vi "Copy .LLB to NI VeriStand dir.vi"(5 "Files Generated by Build":path[](array[path]), 6 "Top Level/Always Included VIs":path[](array[path]), 7 "Destination Path":path, 8 "error in (no error)":errorcluster, 9 "Target Name":string, 10 "Build Specification Name":string, 11 "Project Path":path) -> (0 "error out":errorcluster)   [LabVIEW 2017]
doc: "This VI is called after each run of a build specification. The VI will copy the generated LLB (Engine or System Explorer) into the VeriStand Custom Device folder (...\\Documents\\National Instruments\\NI VeriStand 2013...)."
uses:
  <vilib>/Utility/sysdir.llb/System Directory Type.ctl
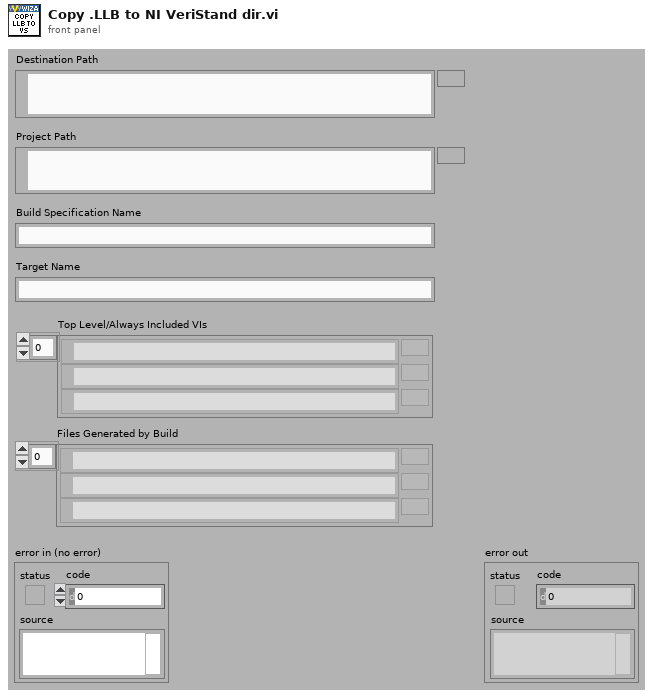
[diagram p1: front panel]
types:
  T1 = typedef "System Directory Type.ctl" = i32
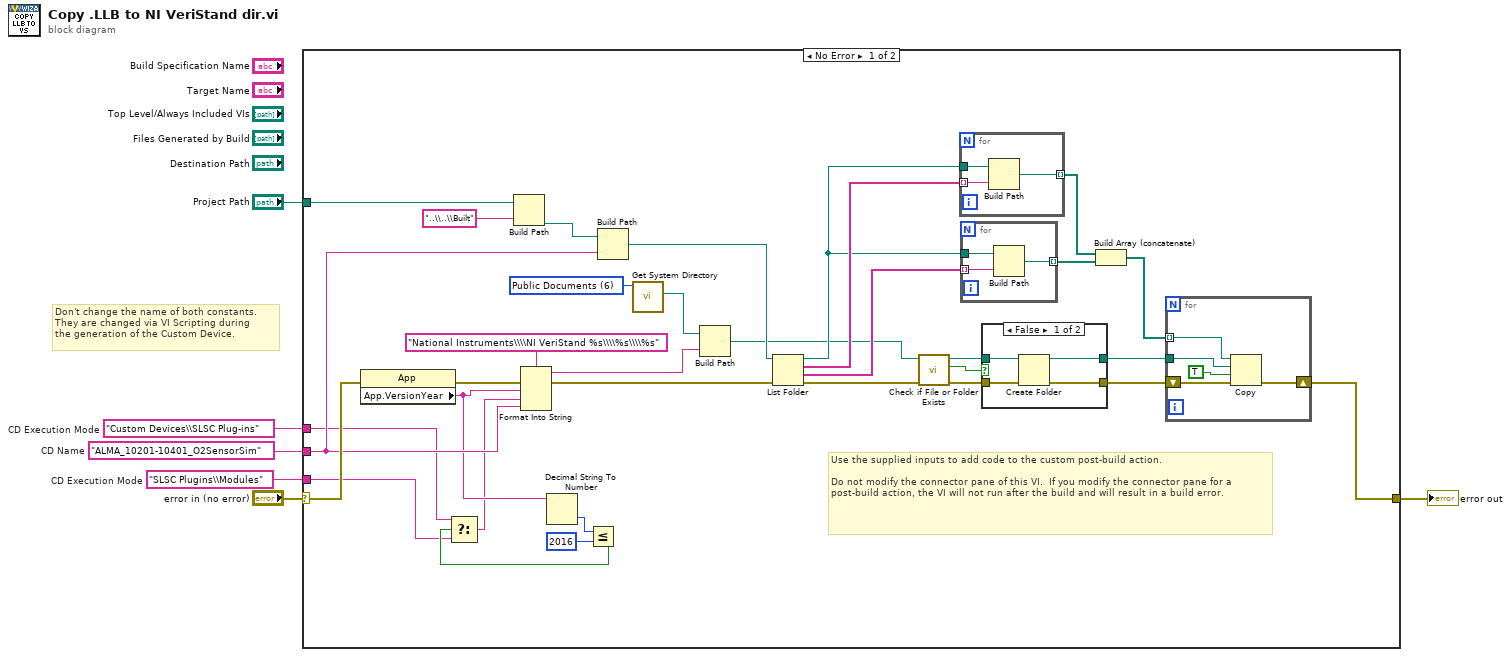
[diagram p0: block diagram]
diagram:
  w1 = "SLSC Plugins\\Modules"  # CD Execution Mode
  w3 = "ALMA_10201-10401_O2SensorSim"  # CD Name
  w4 = "Custom Devices\\SLSC Plug-ins"  # CD Execution Mode
  # "Don't change the name of both constants.\nThey are changed via VI Scripting during\nthe generation of the Custom Device."
  n1 = case shown="No Error" "error in (no error)" {
    selector: "error in (no error)" -> [w20 w57]
    tunnel: [w22 w57] -> w2
    tunnel: "Project Path" -> [w16 _]
    tunnel: w4 -> [w8 _]
    tunnel: w3 -> [w18 _]
    tunnel: w1 -> [w7 _]
    frame No Error {
      w25 = T1 6 items=["User Home"=0, "User Desktop"=1, "User Documents"=2, "User Application Data"=3, "User Preferences"=4, "User Temporary"=5, "Public Documents"=6, "Public Application Data"=7, "Public Preferences"=8, "Public Cache"=13, "System Core Libraries"=9, "System Installed Libraries"=10, "Application Files"=11, "Boot Volume Root"=12] ("system directory type")
      # "Use the supplied inputs to add code to the custom post-build action.\n\nDo not modify the connector pane of this VI.  If you modify the connector pane for a post-build action, the VI will not run after the build and will result in a build error."
      n2 = property class="App"(error in=w20) -> (error out=w24:errorcluster, "App.VersionYear"=w13:string)  [unwired: 1 in, 1 out]
      n3 = Build Path(base path=w16, name or relative path="..\\..\\Built") -> (appended path=w28:path)
      n4 = Decimal String To Number(string=w13) -> (number=w12:i32)  [unwired: 2 in, 1 out]
      n5 = Less Or Equal?(x=w12, y=2016) -> (x <= y?=w10:bool)
      n6 = Select(t=w8, s=w10, f=w7) -> (s? t:f=w9:string)
      n7 = Format Into String(format string="National Instruments\\\\NI VeriStand %s\\\\%s\\\\%s" ("name or relative path"), error in=w24, w13, w9, w18) -> (resulting string=w27:string, error out=w19:errorcluster)  [unwired: 1 in]
      n8 = Build Path(base path=w28, name or relative path=w18) -> (appended path=w30:path)
      n9 = call <vilib>:"Get System Directory.vi"("system directory type"=w25) -> ("system directory"=w26:path)  [unwired: 10 in]
      n10 = Build Path(base path=w26, name or relative path=w27) -> (appended path=w21:path)
      n11 = List Folder(path=w30, error in=w19) -> (path out=w32:path, filenames=w39:string[], folder names=w33:string[], error out=w29:errorcluster)  [unwired: 2 in]
      n12 = call <vilib>:"Check if File or Folder Exists.vi"("error in (no error)"=w29, "path"=w21) -> ("error out"=w34:errorcluster, "file or folder exists?"=w36:bool, "dup path"=w35:path)  [unwired: 7 in]
      n13 = for {
        tunnel: w39 -> [w55] mode=indexing
        tunnel: w32 -> [w56]
        tunnel: [w54] -> w38 mode=indexing
        n14 = Build Path(base path=w56, name or relative path=w55) -> (appended path=w54:path)
      }
      n15 = for {
        tunnel: w33 -> [w52] mode=indexing
        tunnel: w32 -> [w53]
        tunnel: [w51] -> w31 mode=indexing
        n16 = Build Path(base path=w53, name or relative path=w52) -> (appended path=w51:path)
      }
      n17 = case shown="False" w36 {
        tunnel: w35 -> [w43 w45]
        tunnel: w34 -> [w42 w44]
        tunnel: [w41 w45] -> w15
        tunnel: [w40 w44] -> w14
        frame False {
          n18 = Create Folder(path (use dialog)=w43, error in=w42) -> (created path=w41:path, error out=w40:errorcluster)  [unwired: 1 in, 1 out]
        }
        frame True {
        }
      }
      n19 = Build Array (concatenate)(w38, w31) -> (w37:path[])
      n20 = for {
        tunnel: w37 -> [w47] mode=indexing
        shift-right: [w48] -> w22
        shift-left: w14 -> [w49]
        tunnel: w15 -> [w46]
        n21 = Copy(8:w49, 9:TRUE ("overwrite (F)"), 10:w46, 11:w47) -> (0:w48:errorcluster)  [unwired: 1 in, 2 out]
      }
    }
    frame Error {
    }
  }
  "error out" <- w2
